vi "Temp scan setup.vi"(7 "VISA resource name":refnum<visa-resource-name>, 8 "error in (no error)":errorcluster caption="错误输入（无错误）", 9 "数值":i32, 10 "通道":string, 11 "6510 输入":refnum<class "6510.lvclass">) -> (0 "error out":errorcluster caption="错误输出", 3 "6510 输出":refnum<class "6510.lvclass">)   [LabVIEW 2021, in "6510.lvclass"]
uses:
  6510.lvclass
  6510.lvclass/6510.ctl
  <instrlib>/Keithley DMM6500 DAQ6500 Series/Public/Configure/Configure Temperature (Thermocouple).vi
  <instrlib>/Keithley DMM6500 DAQ6500 Series/Keithley DMM6500 DAQ6500 Series.lvlib
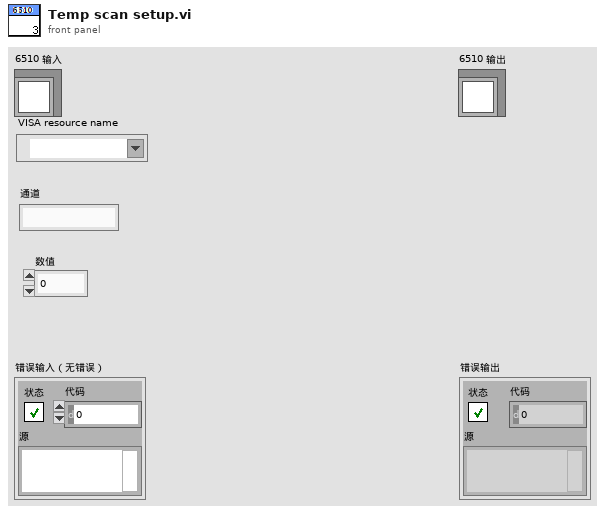
[diagram p1: front panel]
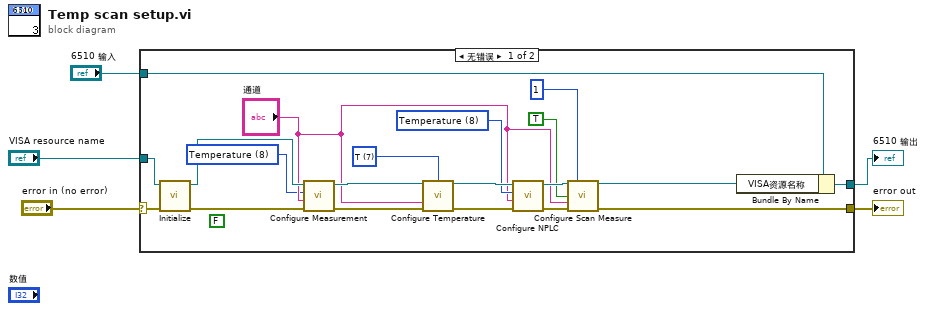
[diagram p0: block diagram]
diagram:
  n1 = case shown="无错误" "error in (no error)" {
    selector: "error in (no error)" -> [w12 w27]
    tunnel: "6510 输入" -> [w9 w26]
    tunnel: [w11 w27] -> w3
    tunnel: [w7 w26] -> w2
    tunnel: "VISA resource name" -> [w10 _]
    frame No Error {
      (unwired) FALSE ("Clear Buffer (No)")
      w13 = 8 items=[" Voltage DC", "Voltage AC", "Current DC", "Current AC", "Resistance", "4-wire Resistance", "Diode", "Capacitance", "Temperature", "Continuity", "Frequency", "Period", "Voltage Ratio"] ("Function (0: Voltage DC)")
      w19 = 8 items=[" Voltage DC"=0, "Current DC"=2, "Resistance"=4, "4-wire Resistance"=5, "Diode"=6, "Temperature"=8, "Voltage Ratio"=12] ("Function (0: Voltage DC)")
      w21 = 7 items=["B", "E", "J", "K", "N", "R", "S", "T"] ("Thermocouple Type (3: K)")
      n2 = call <instrlib>:"Initialize.vi"("error in (no error)"=w12, "VISA resource name"=w10) -> ("error out"=w23:errorcluster, "VISA resource name out"=w24:refnum<visa-resource-name>)  [unwired: 8 in]
      n3 = call <instrlib>:"Configure Measurement.vi"("error in (no error)"=w23, "Channel List(\"\")"="通道", "Function (0: Voltage DC)"=w13, "VISA resource name"=w24) -> ("error out"=w22:errorcluster, "VISA resource name out"=w25:refnum<visa-resource-name>)  [unwired: 6 in]
      n4 = call-poly <instrlib>:"Configure Temperature.vi"("VISA resource name"=w25, "Thermocouple Type (3: K)"=w21, "Channel List(\"\")"="通道", "error in (no error)"=w22) -> ("VISA resource name out"=w20:refnum<visa-resource-name>, "error out"=w18:errorcluster)  [unwired: 10 in]
      n5 = call <instrlib>:"Configure NPLC.vi"("error in (no error)"=w18, "Channel List(\"\")"="通道", "Function (0: Voltage DC)"=w19, "VISA resource name"=w20) -> ("error out"=w15:errorcluster, "VISA resource name out"=w17:refnum<visa-resource-name>)  [unwired: 6 in]
      n6 = call <instrlib>:"Configure Scan Measure.vi"("VISA resource name"=w17, "Scan Count (0)"=u32 1, "Enable Scan Reset (T: Enable)"=TRUE, "Channel List(\"\")"="通道", "error in (no error)"=w15) -> ("VISA resource name out"=w8:refnum<visa-resource-name>, "error out"=w11:errorcluster)  [unwired: 9 in]
      n7 = Bundle By Name(cluster=w9, "VISA资源名称"=w8) -> (w7:refnum<class "6510.lvclass">)
    }
    frame Error {
    }
  }
  "error out" <- w3
  "6510 输出" <- w2
